vi "create default channels.vi"() -> (0 "error out":errorcluster, 1 "tag names":string[](array[string]), 2 "channels":refnum<class "TBM channel.lvclass">[](array[class]), 3 "module":refnum<class "current tag file io module configuration.lvclass">, 5 "instance identifier":string)   [LabVIEW 2013, in "current tag file io module tests.lvlib"]
uses:
  current tag file io module tests.lvlib
  <vilib>/NI/Tag Bus Module Framework/channel/TBM channel.lvclass
  module/configuration/current tag file io module configuration.lvclass
  <vilib>/NI/Tag Bus/tag/Data Type.ctl
  <vilib>/NI/Tag Bus Module Framework/channel/channel classification.ctl
  <vilib>/NI/Tag Bus/tag/tag descriptor.lvclass/tag descriptor.ctl
  <vilib>/NI/Configuration Framework/serializable configuration/NISE_CEF_serializable configuration.lvclass
  <vilib>/NI/Tag Bus/tag/tag descriptor.lvclass
panel:
  in  "Data Type":T1
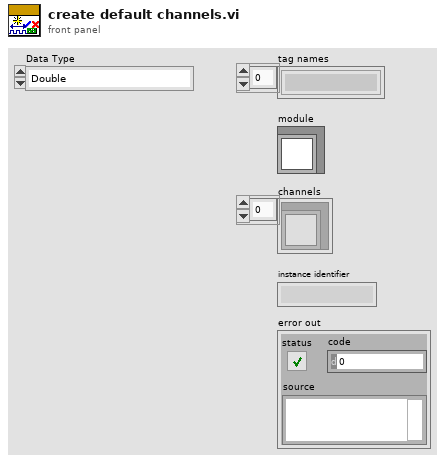
[diagram p1: front panel]
types:
  T1 = typedef "tag bus.lvlib/tag descriptor.lvclass/Data Type.ctl" = enum16{"Double", "Single", "I64", "I32", "I16", "I8", "U64", "U32", "U16", "U8", "Boolean", "String", "Array of Double", "Array of Single", "Array of I64", "Array of I32", "Array of I16", "Array of I8", "Array of U64", "Array of U32", "Array of U16", "Array of U8", "Array of Boolean", "Array of String"}
  T2 = typedef "TBM channel.lvclass/channel classification.ctl" = enum16{"input data", "output data", "processing parameter", "processing result"}
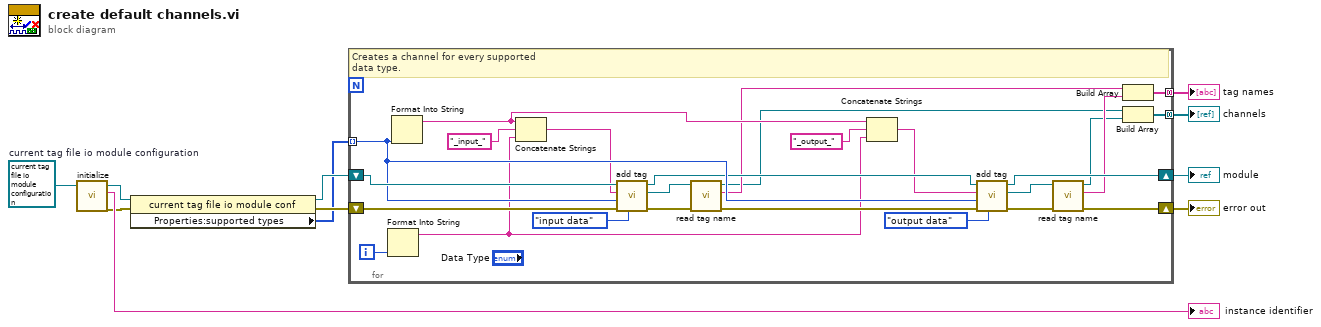
[diagram p0: block diagram]
diagram:
  w3 = refnum<class "current tag file io module configuration.lvclass"> refnum  # current tag file io module configuration
  n1 = call <vilib>:"initialize.vi"("configuration in"=w3) -> ("error out"=w9:errorcluster, "identifier"=→"instance identifier":string, "configuration out"=w7:refnum<class "current tag file io module configuration.lvclass">)  [unwired: 8 in]
  n2 = property class="current tag file io module conf"(reference=w7, error in=w9) -> (reference out=w5:refnum<class "current tag file io module configuration.lvclass">, error out=w8:errorcluster, "Properties:supported types"=w4:T1[])
  n3 = for {
    shift-right: [w33] -> w6
    shift-left: w5 -> [w36]
    shift-right: [w26] -> w11
    shift-left: w8 -> [w37]
    tunnel: w4 -> [w35] mode=indexing
    tunnel: [w12] -> w1 mode=concatenating
    tunnel: [w15] -> w2 mode=concatenating
    i -> [w22]
    # "Creates a channel for every supported\ndata type."
    n4 = Format Into String(w22) -> (resulting string=w19:string)  [unwired: 3 in, 1 out]
    n5 = Format Into String(w35) -> (resulting string=w20:string)  [unwired: 3 in, 1 out]
    n6 = Concatenate Strings(w20, "_input_" ("string"), w19) -> (w24:string)
    n7 = call "add tag.vi"("channel classification (input data)"=channel_classification."input data", "error in"=w37, "data type"=w35, "tag name"=w24, "current tag file io module configuration in"=w36) -> ("error out"=w29:errorcluster, "created channel"=w30:refnum<class "TBM channel.lvclass">, "current tag file io module configuration out"=w34:refnum<class "current tag file io module configuration.lvclass">)  [unwired: 4 in]
    n8 = call <vilib>:"read tag name.vi"("error in"=w29, "system tag in"=w30) -> ("error out"=w28:errorcluster, "name"=w17:string, "system tag out"=w14:refnum<class "TBM channel.lvclass">)  [unwired: 7 in]
    n9 = Concatenate Strings(w20, "_output_" ("string"), w19) -> (w18:string)
    n10 = call "add tag.vi"("channel classification (input data)"=channel_classification."output data", "error in"=w28, "data type"=w35, "tag name"=w18, "current tag file io module configuration in"=w34) -> ("error out"=w27:errorcluster, "created channel"=w25:refnum<class "TBM channel.lvclass">, "current tag file io module configuration out"=w33:refnum<class "current tag file io module configuration.lvclass">)  [unwired: 4 in]
    n11 = call <vilib>:"read tag name.vi"("error in"=w27, "system tag in"=w25) -> ("error out"=w26:errorcluster, "name"=w16:string, "system tag out"=w13:refnum<class "TBM channel.lvclass">)  [unwired: 7 in]
    n12 = Build Array(w17, w16) -> (w15:string[])
    n13 = Build Array(w14, w13) -> (w12:refnum<class "TBM channel.lvclass">[])
  }
  "error out" <- w11
  "channels" <- w1
  "module" <- w6
  "tag names" <- w2
